vi "Polynomial Eigenvalue Problem (DBL, Genl Case).vi"(10 "output option":i32(ring)=1 items=["eigenvalues", "eigenvalues & vectors"], 11 "Input Matrices":dbl[][][](array[numeric])) -> (0 "error":i32, 2 "Eigenvectors":T1, 3 "Eigenvalues":cdb[](array[numeric]))   [LabVIEW 2020, in "NI_AALPro.lvlib"]
uses:
  NI_AALPro.lvlib
  ComplexMatrix.ctl
  Real Generalized Eigenvalues and Vectors.vi
  Create Special Real Matrix.vi
  NI_Matrix.lvlib
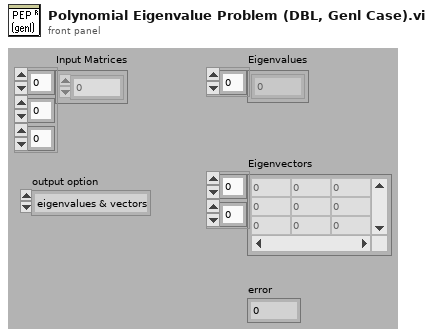
[diagram p1: front panel]
types:
  T1 = typedef "NI_Matrix.lvlib/ComplexMatrix.ctl" = cdb[][]
  T2 = enum32{"Identity", "Diagonal", "Toepliz", "Vandermonde", "Companion"}
  T3 = typedef "NI_Matrix.lvlib/RealMatrix.ctl" = dbl[][]
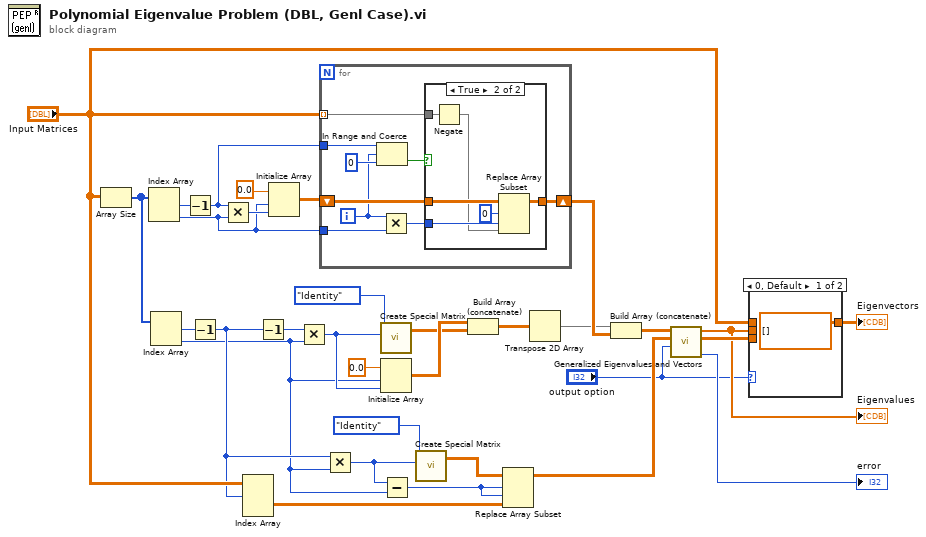
[diagram p0: block diagram]
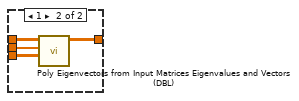
[diagram p2: hidden frame]
diagram:
  n1 = Array Size(array="Input Matrices") -> (size(s)=w26:i32[])
  n2 = Index Array(array=w26) -> (element #1=w18:i32, element #2=w29:i32)  [unwired: 2 in]
  n3 = Index Array(array=w26) -> (element #1=w19:i32, element #2=w3:i32)  [unwired: 2 in]
  n4 = Decrement(x=w18) -> (x-1=w17:i32)
  n5 = Decrement(x=w19) -> (x-1=w4:i32)
  n6 = Multiply(x=w17, y=w29) -> (x*y=w32:i32)
  n7 = Index Array(array="Input Matrices", index (dim 0)=w4) -> (element=w23:dbl[][])  [unwired: 2 in]
  n8 = Decrement(x=w4) -> (x-1=w20:i32)
  n9 = Initialize Array(0.0, w29, w32) -> (w30:dbl[][])
  n10 = Multiply(x=w20, y=w3) -> (x*y=w22:i32)
  n11 = for {
    shift-right: [w36] -> w8
    shift-left: w30 -> [w38]
    tunnel: "Input Matrices" -> [w37] mode=indexing
    tunnel: w17 -> [w40]
    tunnel: w29 -> [w35]
    i -> [w33]
    n12 = In Range and Coerce(upper limit=w40, x=w33, lower limit=0) -> (In Range?=w39:bool)  [unwired: 1 out]
    n13 = Multiply(x=w33, y=w35) -> (x*y=w34:i32)
    n14 = case shown="True" w39 {
      tunnel: w38 -> [w42 w48]
      tunnel: [w42 w47] -> w36
      tunnel: w37 -> [_ w44]
      tunnel: w34 -> [_ w45]
      frame False {
      }
      frame True {
        n15 = Negate(x=w44) -> (-x=w43:dbl[][])
        n16 = Replace Array Subset(array=w48, new element=w43, index (row)=0, index (col)=w45) -> (w47:dbl[][])
      }
    }
  }
  n17 = Multiply(x=w4, y=w3) -> (x*y=w11:i32)
  n18 = call-poly "Create Special Matrix.vi"("matrix type"=T2."Identity", "matrix size"=w22) -> ("Special Matrix"=w5:T3)  [unwired: 3 in, 1 out]
  n19 = Initialize Array(0.0 ("element"), w3, w22) -> (w6:dbl[][])
  n20 = Subtract(x=w11, y=w3) -> (x-y=w12:i32)
  n21 = call-poly "Create Special Matrix.vi"("matrix type"=T2."Identity", "matrix size"=w11) -> ("Special Matrix"=w24:T3)  [unwired: 3 in, 1 out]
  n22 = Build Array (concatenate)(w6, w5) -> (w21:T3)
  n23 = Replace Array Subset(array=w24, new element=w23, index (row)=w12, index (col)=w12) -> (w9:T3)
  n24 = Transpose 2D Array(2D array=w21) -> (transposed array=w7:T3)
  n25 = Build Array (concatenate)(w7, w8) -> (w10:T3)
  n26 = call-poly "Generalized Eigenvalues and Vectors.vi"("output option"="output option", "B"=w9, "A"=w10) -> ("error"=→"error":i32, "Eigenvectors"=w16:T1, "Eigenvalues"=w13:cdb[])  [unwired: 3 in]
  "Eigenvalues" <- w13
  n27 = case shown="0, Default" "output option" {
    tunnel: w16 -> [_ w53]
    tunnel: "Input Matrices" -> [_ w52]
    tunnel: [T1 [] ("Eigenvectors") w51] -> w14
    tunnel: w13 -> [_ w50]
    frame 0, Default {
    }
    frame 1 {
      n28 = call "Poly Eigenvectors from Input Matrices Eigenvalues and Vectors (DBL).vi"("Eigenvectors"=w53, "Eigenvalues"=w50, "Input Matrices"=w52) -> ("X"=w51:T1)  [unwired: 8 in]
    }
  }
  "Eigenvectors" <- w14
